vi "Create_Simple_AO_Signal.vi"(7 "On/OFF":bool, 8 "error in":errorcluster, 9 "Amplitude":dbl=10000.0, 10 "Samples / s (10000)":u32=10000, 11 "Time (s)":dbl=0.1) -> (0 "error out":errorcluster, 3 "Signal":dbl[](array[numeric]))   [LabVIEW 2025]
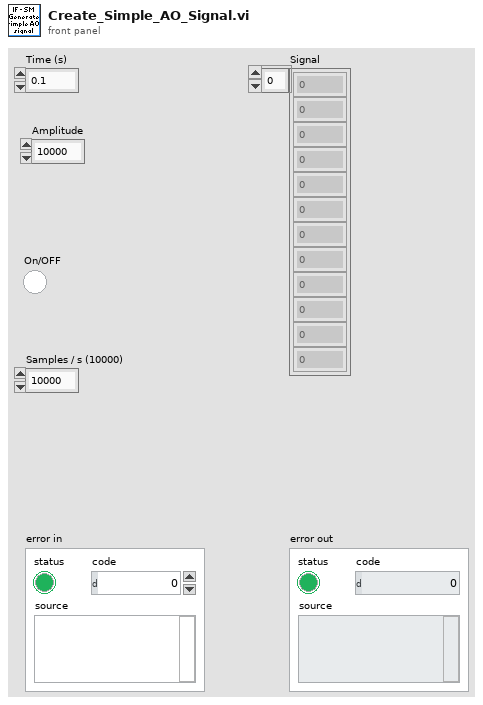
[diagram p1: front panel]
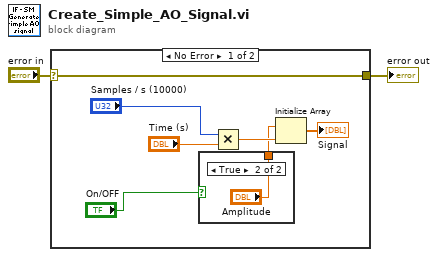
[diagram p0: block diagram]
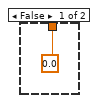
[diagram p2: hidden frame]
diagram:
  n1 = case shown="No Error" "error in" {
    selector: "error in" -> [w6 w12]
    tunnel: [w6 w12] -> w1
    frame No Error {
      n2 = case shown="True" "On/OFF" {
        tunnel: [0.0 ("Amplitude") "Amplitude"] -> w4
        frame False {
        }
        frame True {
        }
      }
      n3 = Multiply(x="Samples / s (10000)", y="Time (s)") -> (x*y=w7:dbl)
      n4 = Initialize Array(w4, w7) -> (→"Signal":dbl[])
    }
    frame Error {
    }
  }
  "error out" <- w1
